vi "FPOpen.vi"(8 "error in (no error)":errorcluster, 11 "VI in":refnum<vi>) -> (0 "error out":errorcluster, 2 "Open?":bool, 3 "VI out":refnum<vi>)   [LabVIEW 2024, in "ModuleManager.lvclass"]
uses:
  ModuleManager.lvclass
  ModuleManager.lvclass/ModuleManager.ctl
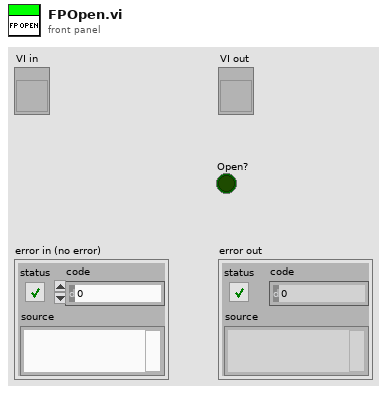
[diagram p1: front panel]
types:
  T1 = enum32{"Invalid", "Standard", "Closed", "Hidden", "Minimized", "Maximized"}
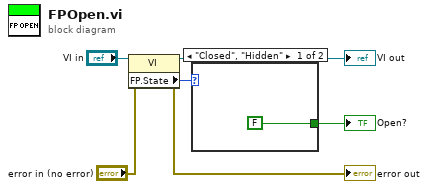
[diagram p0: block diagram]
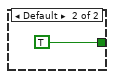
[diagram p2: hidden frame]
diagram:
  n1 = property class="VI"(reference="VI in", error in="error in (no error)") -> (reference out=→"VI out":refnum<vi>, error out=→"error out":errorcluster, "FP.State"=w5:T1)
  n2 = case shown="\"Closed\", \"Hidden\"" w5 {
    tunnel: [FALSE TRUE] -> w6
    frame "Closed", "Hidden" {
    }
    frame Default {
    }
  }
  "Open?" <- w6
